vi "LuaVIEW Parse Function Documentation.vi"(7 "documentation":string) -> (4 "formatting error":string, 8 "unnamed synopsis":string)   [LabVIEW 2012]
doc: "Parses the function documentation and formats a function call synopsis that has a \"%s\" format specifier that allows the function name and optional table to be inserted. If the documentation is malformed, an error is output."
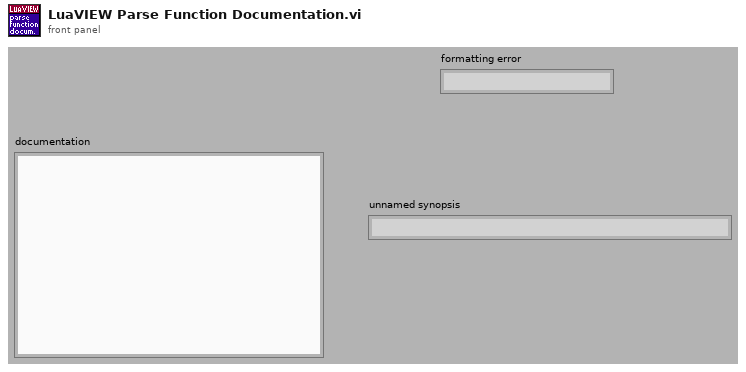
[diagram p1: front panel]
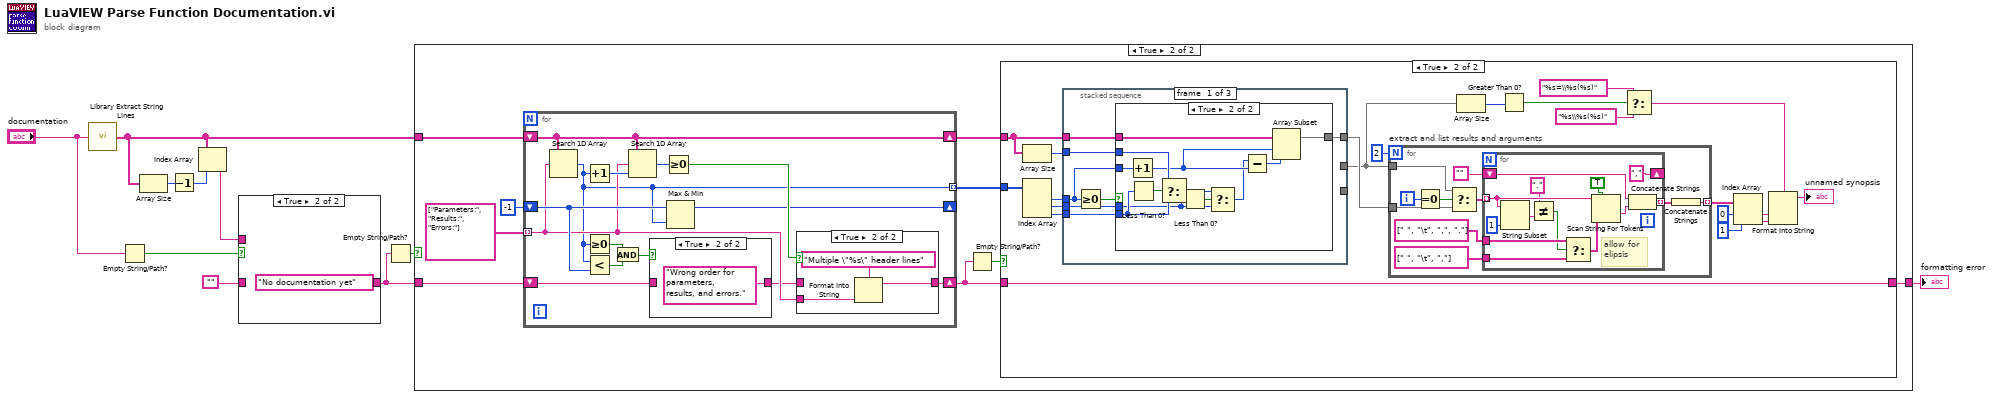
[diagram p0: block diagram]
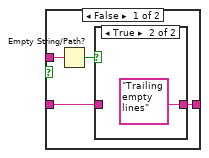
[diagram p2: hidden frame]
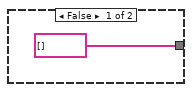
[diagram p6: hidden frame]
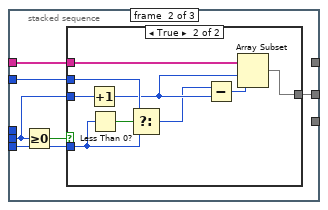
[diagram p7: hidden frame]
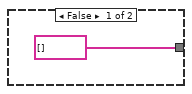
[diagram p8: hidden frame]
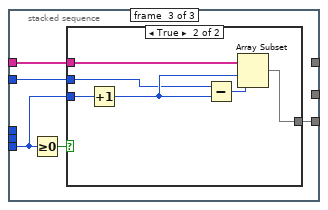
[diagram p9: hidden frame]
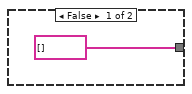
[diagram p10: hidden frame]
diagram:
  n1 = call "Library Extract String Lines.vi"("multi-line string"="documentation") -> ("lines"=w6:string[])  [unwired: 14 in]
  n2 = Empty String/Path?(string/path="documentation") -> (empty?=w9:bool)
  n3 = Array Size(array=w6) -> (size(s)=w7:i32)
  n4 = Decrement(x=w7) -> (x-1=w5:i32)
  n5 = Index Array(array=w6, index=w5) -> (element=w2:string)
  n6 = case shown="True" w9 {
    tunnel: "" -> [w13 _]
    tunnel: [w11 "No documentation yet"] -> w4
    tunnel: w2 -> [w14 _]
    frame False {
      n7 = Empty String/Path?(string/path=w14) -> (empty?=w12:bool)
      n8 = case shown="True" w12 {
        tunnel: w13 -> [w15 _]
        tunnel: [w15 "Trailing empty lines"] -> w11
        frame False {
        }
        frame True {
        }
      }
    }
    frame True {
    }
  }
  n9 = Empty String/Path?(string/path=w4) -> (empty?=w3:bool)
  n10 = case shown="True" w3 {
    tunnel: w6 -> [_ w27]
    tunnel: [w18 w20] -> w1
    tunnel: w4 -> [w18 w19]
    frame False {
    }
    frame True {
      n11 = for {
        shift-right: [w134] -> w23
        shift-left: w27 -> [w134]
        tunnel: string[] ["Parameters:", "Results:", "Errors:"] -> [w127] mode=indexing
        tunnel: [w124] -> w24 mode=indexing
        shift-right: [w131] -> w21
        shift-left: w19 -> [w126]
        shift-right: [w128] -> _
        shift-left: -1 -> [w129]
        n12 = Search 1D Array(1D array=w134, element=w127) -> (index of element=w124:i32)  [unwired: 1 in]
        n13 = Increment(x=w124) -> (x+1=w130:i32)
        n14 = Greater Or Equal To 0?(x=w124) -> (x >= 0?=w123:bool)
        n15 = Less?(x=w124, y=w129) -> (x < y?=w122:bool)
        n16 = And(x=w123, y=w122) -> (x .and. y?=w121:bool)
        n17 = Search 1D Array(1D array=w134, element=w127, start index (0)=w130) -> (index of element=w133:i32)
        n18 = case shown="True" w121 {
          tunnel: w126 -> [w135 _]
          tunnel: [w135 "Wrong order for parameters, results, and errors."] -> w125
          frame False {
          }
          frame True {
          }
        }
        n19 = Greater Or Equal To 0?(x=w133) -> (x >= 0?=w132:bool)
        n20 = Max & Min(x=w129, y=w124) -> (max(x,y)=w128:i32)  [unwired: 1 out]
        n21 = case shown="True" w132 {
          tunnel: [w137 w140] -> w131
          tunnel: w125 -> [w137 _]
          tunnel: w127 -> [_ w139]
          frame False {
          }
          frame True {
            n22 = Format Into String(format string="Multiple \"%s\" header lines", w139) -> (resulting string=w140:string)  [unwired: 2 in, 1 out]
          }
        }
      }
      n23 = Empty String/Path?(string/path=w21) -> (empty?=w22:bool)
      n24 = case shown="True" w22 {
        tunnel: w24 -> [_ w49]
        tunnel: w23 -> [_ w44]
        tunnel: w21 -> [w28 w36]
        tunnel: [w28 w36] -> w20
        frame False {
        }
        frame True {
          n25 = Array Size(array=w44) -> (size(s)=w48:i32)
          n26 = Index Array(array=w49) -> (element #1=w47:i32, element #2=w46:i32, element #3=w45:i32)  [unwired: 3 in]
          n27 = stacked-sequence {
            tunnel: w48 -> [w76 w96 w111]
            tunnel: w47 -> [w73 _ _]
            tunnel: w46 -> [w75 w93 _]
            tunnel: w45 -> [w74 w95 w110]
            tunnel: [w78 _ _] -> w43
            tunnel: w44 -> [w77 w97 w112]
            tunnel: [_ w94 _] -> w34
            tunnel: [_ _ w109] -> _
            frame #0 {
              n28 = Greater Or Equal To 0?(x=w73) -> (x >= 0?=w79:bool)
              n29 = case shown="True" w79 {
                tunnel: [string[] [] ("lines") w81] -> w78
                tunnel: w77 -> [_ w85]
                tunnel: w76 -> [_ w92]
                tunnel: w75 -> [_ w87]
                tunnel: w74 -> [_ w88]
                tunnel: w73 -> [_ w86]
                frame False {
                }
                frame True {
                  n30 = Increment(x=w86) -> (x+1=w84:i32)
                  n31 = Less Than 0?(x=w88) -> (x < 0?=w91:bool)
                  n32 = Select(t=w92, s=w91, f=w88) -> (s? t:f=w90:i32)
                  n33 = Less Than 0?(x=w87) -> (x < 0?=w89:bool)
                  n34 = Select(t=w90, s=w89, f=w87) -> (s? t:f=w83:i32)
                  n35 = Subtract(x=w83, y=w84) -> (x-y=w82:i32)
                  n36 = Array Subset(array=w85, index=w84, length=w82) -> (w81:string[])
                }
              }
            }
            frame #1 {
              n37 = Greater Or Equal To 0?(x=w93) -> (x >= 0?=w98:bool)
              n38 = case shown="True" w98 {
                tunnel: [string[] [] ("lines") w102] -> w94
                tunnel: w97 -> [_ w104]
                tunnel: w96 -> [_ w108]
                tunnel: w95 -> [_ w106]
                tunnel: w93 -> [_ w105]
                frame False {
                }
                frame True {
                  n39 = Increment(x=w105) -> (x+1=w101:i32)
                  n40 = Less Than 0?(x=w106) -> (x < 0?=w107:bool)
                  n41 = Select(t=w108, s=w107, f=w106) -> (s? t:f=w100:i32)
                  n42 = Subtract(x=w100, y=w101) -> (x-y=w103:i32)
                  n43 = Array Subset(array=w104, index=w101, length=w103) -> (w102:string[])
                }
              }
            }
            frame #2 {
              n44 = Greater Or Equal To 0?(x=w110) -> (x >= 0?=w113:bool)
              n45 = case shown="True" w113 {
                tunnel: [string[] [] ("lines") w117] -> w109
                tunnel: w112 -> [_ w119]
                tunnel: w111 -> [_ w115]
                tunnel: w110 -> [_ w120]
                frame False {
                }
                frame True {
                  n46 = Increment(x=w120) -> (x+1=w116:i32)
                  n47 = Subtract(x=w115, y=w116) -> (x-y=w118:i32)
                  n48 = Array Subset(array=w119, index=w116, length=w118) -> (w117:string[])
                }
              }
            }
          }
          n49 = for "extract and list results and arguments" {
            N: 2 -> [_]
            tunnel: w43 -> [w54]
            tunnel: w34 -> [w55]
            tunnel: [w53] -> w33 mode=indexing
            i -> [w57]
            n50 = Equal To 0?(x=w57) -> (x = 0?=w56:bool)
            n51 = Select(t=w55, s=w56, f=w54) -> (s? t:f=w52:string[])
            n52 = for {
              tunnel: w52 -> [w67] mode=indexing
              shift-right: [","] -> _
              shift-left: "" -> [w70]
              tunnel: [w71] -> w58 mode=indexing
              tunnel: string[] [" ", "\t", ",", "."] ("delimiters (\\s,\\t,\\r,\\n)") -> [w65]
              tunnel: string[] [" ", "\t", ","] ("delimiters (\\s,\\t,\\r,\\n)") -> [w60]
              # "allow for\nelipsis"
              n53 = String Subset(string=w67, length (rest)=1 ("length (rest)")) -> (substring=w64:string)  [unwired: 1 in]
              n54 = Not Equal?(x="." ("y"), y=w64) -> (x != y?=w62:bool)
              n55 = Select(t=w65, s=w62, f=w60) -> (s? t:f=w61:string[])
              n56 = Scan String For Tokens(5:TRUE ("allow empty tokens? (F)"), 6:w61, 9:w67) -> (1:w68:string)  [unwired: 3 in, 3 out]
              n57 = Concatenate Strings(w70, w68) -> (w71:string)
            }
            n58 = Concatenate Strings(w58) -> (w53:string)
          }
          n59 = Array Size(array=w34) -> (size(s)=w41:i32)
          n60 = Greater Than 0?(x=w41) -> (x > 0?=w40:bool)
          n61 = Select(t="%s=\\%s(%s)" ("format string"), s=w40, f="%s\\%s(%s)" ("format string")) -> (s? t:f=w38:string)
          n62 = Index Array(array=w33, index #1=0 ("index"), index #2=1 ("index")) -> (element #1=w30:string, element #2=w29:string)
          n63 = Format Into String(format string=w38, w30, w29) -> (resulting string=→"unnamed synopsis":string)  [unwired: 2 in, 1 out]
        }
      }
    }
  }
  "formatting error" <- w1
